vi "Dictionary.vi"(0 "Variant_In":variant, 5 "Key":string, 11 "error in (no error)":errorcluster, 13 "Dictionary States":T1) -> (4 "Variant_Out":variant, 15 "error out":errorcluster)   [LabVIEW 2021, in "Dictionary.lvlib"]
uses:
  Dictionary.lvlib
  controls/Dictionary States.ctl
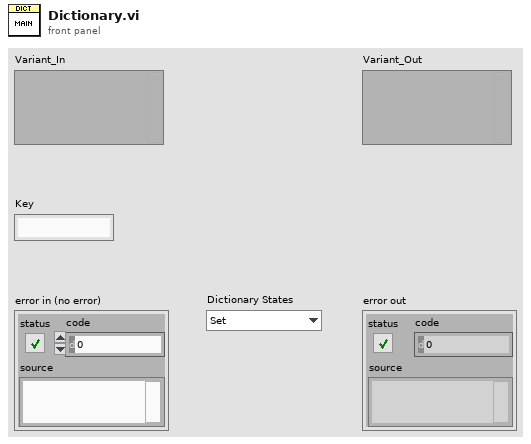
[diagram p1: front panel]
types:
  T1 = typedef "Dictionary.lvlib/Dictionary States.ctl" = enum16{"Set", "Get", "Delete", "Delete All"}
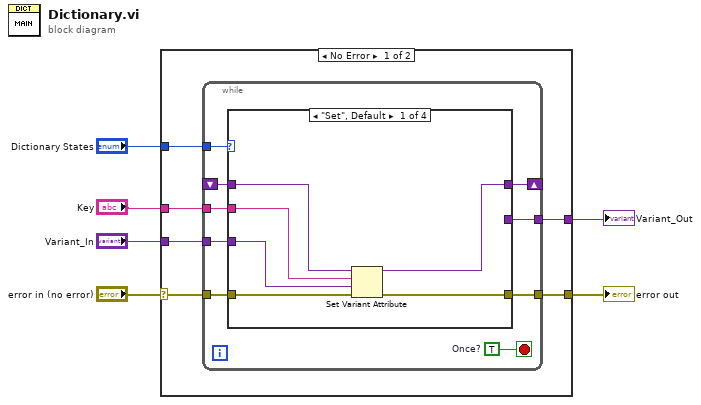
[diagram p0: block diagram]
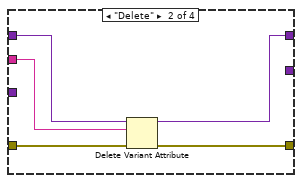
[diagram p2: hidden frame]
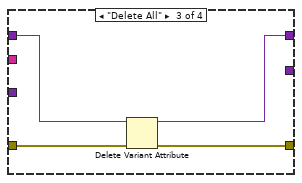
[diagram p3: hidden frame]
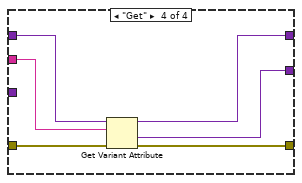
[diagram p4: hidden frame]
diagram:
  n1 = case shown="No Error" "error in (no error)" {
    selector: "error in (no error)" -> [w8 w43]
    tunnel: "Variant_In" -> [w12 _]
    tunnel: "Key" -> [w11 _]
    tunnel: [w10 _] -> w6
    tunnel: "Dictionary States" -> [w9 _]
    tunnel: [w7 w43] -> w2
    frame No Error {
      n2 = while {
        shift-right: [w20] -> _
        shift-left: _ -> [w21]
        tunnel: w12 -> [w19]
        tunnel: w11 -> [w18]
        tunnel: [w17] -> w10
        tunnel: w9 -> [w16]
        tunnel: w8 -> [w15]
        tunnel: [w14] -> w7
        stop <- w13 stop-if-true
        w13 = TRUE  # Once?
        n3 = case shown="\"Set\", Default" w16 {
          tunnel: w21 -> [w27 w32 w36 w42]
          tunnel: [w25 w31 w35 w41] -> w20
          tunnel: w19 -> [w26 _ _ _]
          tunnel: w18 -> [w24 w30 _ w39]
          tunnel: [_ _ _ w40] -> w17
          tunnel: w15 -> [w23 w29 w34 w38]
          tunnel: [w22 w28 w33 w37] -> w14
          frame "Set", Default {
            n4 = Set Variant Attribute(Variant=w27, name=w24, value=w26, error in=w23) -> (Variant out=w25:variant, error out=w22:errorcluster)  [unwired: 1 out]
          }
          frame "Delete" {
            n5 = Delete Variant Attribute(4:w29, 6:w30, 7:w32) -> (0:w28:errorcluster, 3:w31:variant)  [unwired: 1 out]
          }
          frame "Delete All" {
            n6 = Delete Variant Attribute(4:w34, 7:w36) -> (0:w33:errorcluster, 3:w35:variant)  [unwired: 1 in, 1 out]
          }
          frame "Get" {
            n7 = Get Variant Attribute(Variant=w42, name=w39, error in=w38) -> (duplicate Variant=w41:variant, value=w40:variant, error out=w37:errorcluster)  [unwired: 1 in, 1 out]
          }
        }
      }
    }
    frame Error {
    }
  }
  "error out" <- w2
  "Variant_Out" <- w6
